vi "ZK HAL.vi"(11 "Interface":T1={"SYSTEM Interface"={"运行模式"=enum."维护模式", "站点类型"=enum."一体站", "CODMn类型"=enum."PLC版", "总磷总氮类型"=enum."单模块", "CODcr模块版本"=enum."斯坦道V3", "性能测试模式"=FALSE}, "Pump Interface"={"Pump MB session in"=refnum}, "NH3N Interface"={"NH3N session in"=refnum, "氨氮自动测试量程配置"={"水样测试量程模式"=enum."AUTO", "空白核查量程模式"=enum."AUTO", "跨度核查量程模式"=enum."AUTO", "加标回收量程模式"=enum."AUTO"}, "命令格式"=0}, "TP Interface"={"TP MB session in"=refnum, "总磷自动测试量程配置"={"水样测试量程模式"=enum."AUTO", "空白核查量程模式"=enum."AUTO", "跨度核查量程模式"=enum."AUTO", "加标回收量程模式"=enum."AUTO"}, "命令格式"=0}, "TN Interface"={"TN MB session in"=refnum, "总氮自动测试量程配置"={"水样测试量程模式"=enum."AUTO", "空白核查量程模式"=enum."AUTO", "跨度核查量程模式"=enum."AUTO", "加标回收量程模式"=enum."AUTO"}, "命令格式"=0}, "CODMn Interface"={"CODMn MB session in"=refnum, "CODMn自动测试量程配置"={"水样测试量程模式"=enum."AUTO", "空白核查量程模式"=enum."AUTO", "跨度核查量程模式"=enum."AUTO", "加标回收量程模式"=enum."AUTO"}, "命令格式"=0}, "CODCr Interface"={"CODCr MB session in"=refnum, "CODCr自动测试量程配置"={"水样测试量程模式"=enum."AUTO", "空白核查量程模式"=enum."AUTO", "跨度核查量程模式"=enum."AUTO", "加标回收量程模式"=enum."AUTO"}, "命令格式"=0}, "PLC_CODMn Interface"={"PLC版_CODMn状态"=0, "PLC版_CODMn测量数据区"={"因子编码"=0, "单位"=0, "标样参考值"=0.0, "水样数据时间"=timestamp(0 s since 1904-01-01), "水样实测值"=0.0, "水样数据标识"="", "标样数据时间"=timestamp(0 s since 1904-01-01), "标样实测值"=0.0, "标样数据标识"="", "空白数据时间"=timestamp(0 s since 1904-01-01), "空白实测值"=0.0, "空白数据标识"="", "零点核查数据时间"=timestamp(0 s since 1904-01-01), "零点核查实测值"=0.0, "零点核查数据标识"="", "跨度核查数据时间"=timestamp(0 s since 1904-01-01), "跨度核查实测值"=0.0, "跨度核查数据标识"="", "加标回收数据时间"=timestamp(0 s since 1904-01-01), "加标回收实测值"=0.0, "加标回收数据标识"="", "平行样数据时间"=timestamp(0 s since 1904-01-01), "平行样实测值"=0.0, "平行样数据标识"=""}}, "氟化物 Interface"={"MB session in"=refnum, "自动测试量程配置"={"水样测试量程模式"=enum."AUTO", "空白核查量程模式"=enum."AUTO", "跨度核查量程模式"=enum."AUTO", "加标回收量程模式"=enum."AUTO"}}, "挥发酚 Interface"={"挥发酚工作状态"=0, "挥发酚 MB session in"=refnum, "挥发酚_测量数据区"={"因子编码"=0, "单位"=0, "标样2参考值"=0.0, "水样数据时间"=timestamp(0 s since 1904-01-01), "水样实测值"=0.0, "水样数据标识"="", "标样2数据时间"=timestamp(0 s since 1904-01-01), "标样2实测值"=0.0, "标样2数据标识"="", "空白数据时间"=timestamp(0 s since 1904-01-01), "空白实测值"=0.0, "空白数据标识"="", "零点核查数据时间"=timestamp(0 s since 1904-01-01), "零点核查实测值"=0.0, "零点核查数据标识"="", "跨度核查数据时间"=timestamp(0 s since 1904-01-01), "跨度核查实测值"=0.0, "跨度核查数据标识"="", "加标回收数据时间"=timestamp(0 s since 1904-01-01), "加标回收实测值"=0.0, "加标回收数据标识"="", "平行样数据时间"=timestamp(0 s since 1904-01-01), "平行样实测值"=0.0, "平行样数据标识"="", "标样1参考值"=0.0, "标样1数据时间"=timestamp(0 s since 1904-01-01), "标样1实测值"=0.0, "标样1数据标识"="", "标样核查数据时间"=timestamp(0 s since 1904-01-01), "标样核查实测值"=0.0, "标样核查数据标识"=""}}} {"挥发酚 Interface"."挥发酚_测量数据区"."单位" items=["ug/L", "mg/L", "ppm", "mg/m3", "cm", "ppb", "ug/m3", "%", "nmol/mol", "umol/mol", "MPN/L", "MPN/100ml", "ng/m3", "NTU", "无量纲", "ms/cm", "us/cm", "℃", "mV", "万个/L"]; "挥发酚 Interface"."挥发酚工作状态" items=["空闲"=0, "水样测试"=1, "标样核查"=2, "零点核查"=3, "跨度核查"=4, "空白测试"=5, "平行样测试"=6, "加标回收"=7, "空白校准"=8, "标样校准"=9, "标定"=19, "初始化（清洗）"=10, "标样1测量"=28, "标样2测量"=29, "故障"=30, "异常处理"=31, "初始装液"=32, "其他"=33]; "PLC_CODMn Interface"."PLC版_CODMn状态" items=["待机", "润洗", "进样", "加草酸钠", "反滴定", "排液"]; "PLC_CODMn Interface"."PLC版_CODMn测量数据区"."单位" items=["ug/L", "mg/L", "ppm", "mg/m3", "cm", "ppb", "ug/m3", "%", "nmol/mol", "umol/mol", "MPN/L", "MPN/100ml", "ng/m3", "NTU", "无量纲", "ms/cm", "us/cm", "℃", "mV", "万个/L"]; "CODCr Interface"."命令格式" items=["自动", "低位在前", "低位在后"]; "CODMn Interface"."命令格式" items=["自动", "低位在前", "低位在后"]; "TN Interface"."命令格式" items=["自动", "低位在前", "低位在后"]; "TP Interface"."命令格式" items=["自动", "低位在前", "低位在后"]; "NH3N Interface"."命令格式" items=["自动", "低位在前", "低位在后"]}) -> ()   [LabVIEW 2016]
uses:
  <vilib>/Plasmionique/MB Master/MB_Master/MB_Master.lvclass
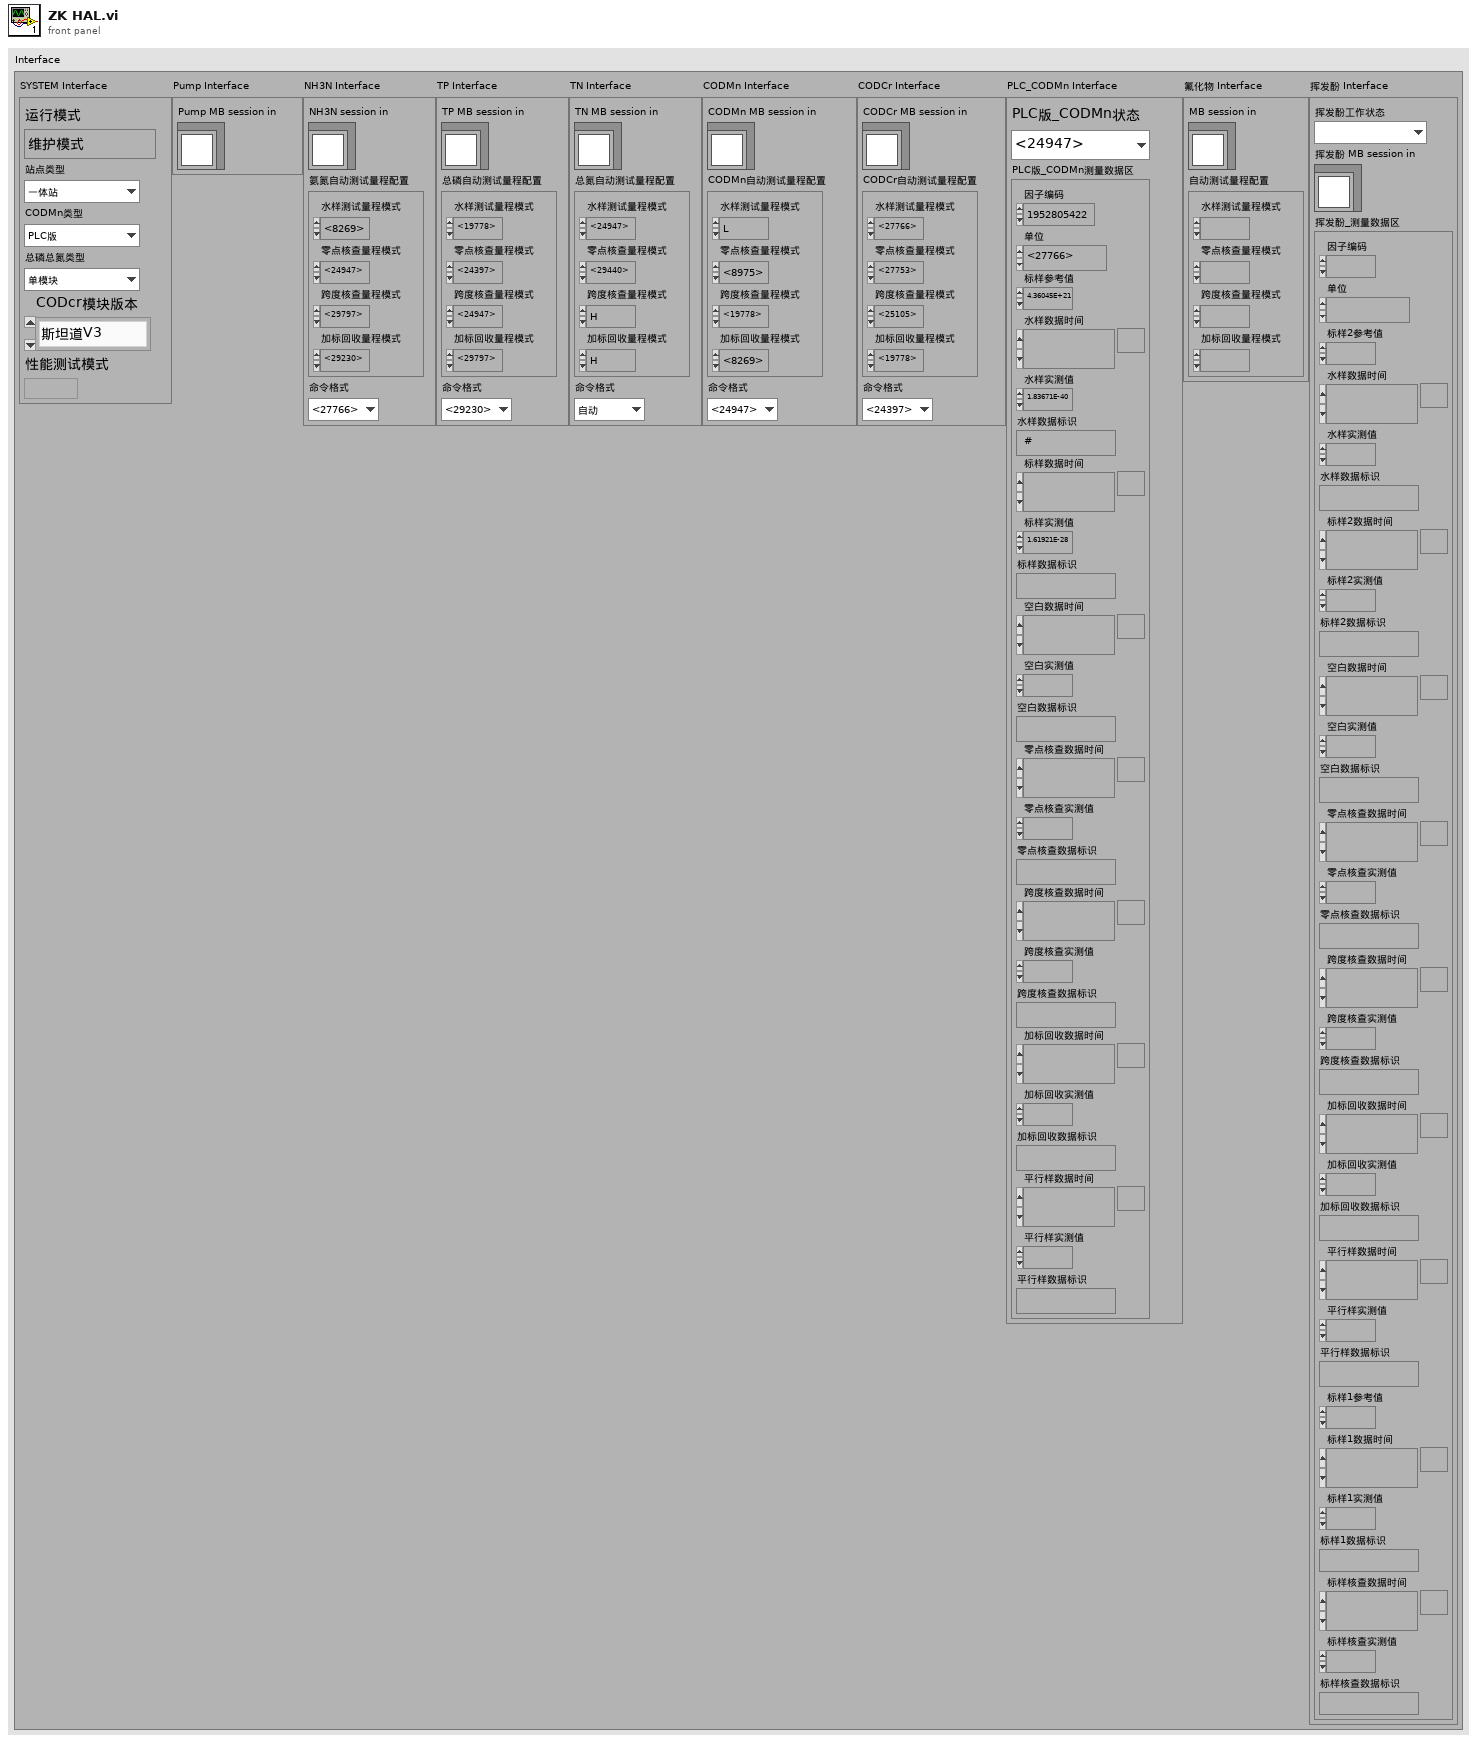
[diagram p1: front panel]
types:
  T1 = cluster{"SYSTEM Interface":cluster{"运行模式":enum16{"维护模式", "常规模式", "应急模式", "质控模式"}, "站点类型":enum16{"一体站", "固定站", "浮船", "一体站V1-V3", "养殖渭水"}, "CODMn类型":enum16{"PLC版", "单片机版"}, "总磷总氮类型":enum16{"单模块", "总磷总氮二合一模块", "氨氮总磷二合一模块"}, "CODcr模块版本":enum16{"斯坦道V3", "点创"}, "性能测试模式":bool}, "Pump Interface":cluster{"Pump MB session in":refnum<class "MB_Master.lvclass">}, "NH3N Interface":cluster{"NH3N session in":refnum<class "MB_Master.lvclass">, "氨氮自动测试量程配置":cluster{"水样测试量程模式":enum16{"H", "L", "AUTO"}, "空白核查量程模式":enum16{"H", "L", "AUTO"}, "跨度核查量程模式":enum16{"H", "L", "AUTO"}, "加标回收量程模式":enum16{"H", "L", "AUTO"}}, "命令格式":u16}, "TP Interface":cluster{"TP MB session in":refnum<class "MB_Master.lvclass">, "总磷自动测试量程配置":cluster{"水样测试量程模式":enum16{"H", "L", "AUTO"}, "空白核查量程模式":enum16{"H", "L", "AUTO"}, "跨度核查量程模式":enum16{"H", "L", "AUTO"}, "加标回收量程模式":enum16{"H", "L", "AUTO"}}, "命令格式":u16}, "TN Interface":cluster{"TN MB session in":refnum<class "MB_Master.lvclass">, "总氮自动测试量程配置":cluster{"水样测试量程模式":enum16{"H", "L", "AUTO"}, "空白核查量程模式":enum16{"H", "L", "AUTO"}, "跨度核查量程模式":enum16{"H", "L", "AUTO"}, "加标回收量程模式":enum16{"H", "L", "AUTO"}}, "命令格式":u16}, "CODMn Interface":cluster{"CODMn MB session in":refnum<class "MB_Master.lvclass">, "CODMn自动测试量程配置":cluster{"水样测试量程模式":enum16{"H", "L", "AUTO"}, "空白核查量程模式":enum16{"H", "L", "AUTO"}, "跨度核查量程模式":enum16{"H", "L", "AUTO"}, "加标回收量程模式":enum16{"H", "L", "AUTO"}}, "命令格式":u16}, "CODCr Interface":cluster{"CODCr MB session in":refnum<class "MB_Master.lvclass">, "CODCr自动测试量程配置":cluster{"水样测试量程模式":enum16{"H", "L", "AUTO"}, "空白核查量程模式":enum16{"H", "L", "AUTO"}, "跨度核查量程模式":enum16{"H", "L", "AUTO"}, "加标回收量程模式":enum16{"H", "L", "AUTO"}}, "命令格式":u16}, "PLC_CODMn Interface":cluster{"PLC版_CODMn状态":u16, "PLC版_CODMn测量数据区":cluster{"因子编码":u32, "单位":u16, "标样参考值":sgl, "水样数据时间":timestamp, "水样实测值":sgl, "水样数据标识":string, "标样数据时间":timestamp, "标样实测值":sgl, "标样数据标识":string, "空白数据时间":timestamp, "空白实测值":sgl, "空白数据标识":string, "零点核查数据时间":timestamp, "零点核查实测值":sgl, "零点核查数据标识":string, "跨度核查数据时间":timestamp, "跨度核查实测值":sgl, "跨度核查数据标识":string, "加标回收数据时间":timestamp, "加标回收实测值":sgl, "加标回收数据标识":string, "平行样数据时间":timestamp, "平行样实测值":sgl, "平行样数据标识":string}}, "氟化物 Interface":cluster{"MB session in":refnum<class "MB_Master.lvclass">, "自动测试量程配置":cluster{"水样测试量程模式":enum16{"H", "L", "AUTO"}, "空白核查量程模式":enum16{"H", "L", "AUTO"}, "跨度核查量程模式":enum16{"H", "L", "AUTO"}, "加标回收量程模式":enum16{"H", "L", "AUTO"}}}, "挥发酚 Interface":cluster{"挥发酚工作状态":u16, "挥发酚 MB session in":refnum<class "MB_Master.lvclass">, "挥发酚_测量数据区":cluster{"因子编码":u32, "单位":u16, "标样2参考值":sgl, "水样数据时间":timestamp, "水样实测值":sgl, "水样数据标识":string, "标样2数据时间":timestamp, "标样2实测值":sgl, "标样2数据标识":string, "空白数据时间":timestamp, "空白实测值":sgl, "空白数据标识":string, "零点核查数据时间":timestamp, "零点核查实测值":sgl, "零点核查数据标识":string, "跨度核查数据时间":timestamp, "跨度核查实测值":sgl, "跨度核查数据标识":string, "加标回收数据时间":timestamp, "加标回收实测值":sgl, "加标回收数据标识":string, "平行样数据时间":timestamp, "平行样实测值":sgl, "平行样数据标识":string, "标样1参考值":sgl, "标样1数据时间":timestamp, "标样1实测值":sgl, "标样1数据标识":string, "标样核查数据时间":timestamp, "标样核查实测值":sgl, "标样核查数据标识":string}}}
  T2 = cluster{"运行模式":enum16{"维护模式", "常规模式", "应急模式", "质控模式"}, "站点类型":enum16{"一体站", "固定站", "浮船", "一体站V1-V3", "养殖渭水"}, "CODMn类型":enum16{"PLC版", "单片机版"}, "总磷总氮类型":enum16{"单模块", "总磷总氮二合一模块", "氨氮总磷二合一模块"}, "CODcr模块版本":enum16{"斯坦道V3", "点创"}, "性能测试模式":bool}
  T3 = cluster{"Pump MB session in":refnum<class "MB_Master.lvclass">}
  T4 = cluster{"NH3N session in":refnum<class "MB_Master.lvclass">, "氨氮自动测试量程配置":cluster{"水样测试量程模式":enum16{"H", "L", "AUTO"}, "空白核查量程模式":enum16{"H", "L", "AUTO"}, "跨度核查量程模式":enum16{"H", "L", "AUTO"}, "加标回收量程模式":enum16{"H", "L", "AUTO"}}, "命令格式":u16}
  T5 = cluster{"TP MB session in":refnum<class "MB_Master.lvclass">, "总磷自动测试量程配置":cluster{"水样测试量程模式":enum16{"H", "L", "AUTO"}, "空白核查量程模式":enum16{"H", "L", "AUTO"}, "跨度核查量程模式":enum16{"H", "L", "AUTO"}, "加标回收量程模式":enum16{"H", "L", "AUTO"}}, "命令格式":u16}
  T6 = cluster{"TN MB session in":refnum<class "MB_Master.lvclass">, "总氮自动测试量程配置":cluster{"水样测试量程模式":enum16{"H", "L", "AUTO"}, "空白核查量程模式":enum16{"H", "L", "AUTO"}, "跨度核查量程模式":enum16{"H", "L", "AUTO"}, "加标回收量程模式":enum16{"H", "L", "AUTO"}}, "命令格式":u16}
  T7 = cluster{"CODMn MB session in":refnum<class "MB_Master.lvclass">, "CODMn自动测试量程配置":cluster{"水样测试量程模式":enum16{"H", "L", "AUTO"}, "空白核查量程模式":enum16{"H", "L", "AUTO"}, "跨度核查量程模式":enum16{"H", "L", "AUTO"}, "加标回收量程模式":enum16{"H", "L", "AUTO"}}, "命令格式":u16}
  T8 = cluster{"CODCr MB session in":refnum<class "MB_Master.lvclass">, "CODCr自动测试量程配置":cluster{"水样测试量程模式":enum16{"H", "L", "AUTO"}, "空白核查量程模式":enum16{"H", "L", "AUTO"}, "跨度核查量程模式":enum16{"H", "L", "AUTO"}, "加标回收量程模式":enum16{"H", "L", "AUTO"}}, "命令格式":u16}
  T9 = cluster{"PLC版_CODMn状态":u16, "PLC版_CODMn测量数据区":cluster{"因子编码":u32, "单位":u16, "标样参考值":sgl, "水样数据时间":timestamp, "水样实测值":sgl, "水样数据标识":string, "标样数据时间":timestamp, "标样实测值":sgl, "标样数据标识":string, "空白数据时间":timestamp, "空白实测值":sgl, "空白数据标识":string, "零点核查数据时间":timestamp, "零点核查实测值":sgl, "零点核查数据标识":string, "跨度核查数据时间":timestamp, "跨度核查实测值":sgl, "跨度核查数据标识":string, "加标回收数据时间":timestamp, "加标回收实测值":sgl, "加标回收数据标识":string, "平行样数据时间":timestamp, "平行样实测值":sgl, "平行样数据标识":string}}
  T10 = cluster{"MB session in":refnum<class "MB_Master.lvclass">, "自动测试量程配置":cluster{"水样测试量程模式":enum16{"H", "L", "AUTO"}, "空白核查量程模式":enum16{"H", "L", "AUTO"}, "跨度核查量程模式":enum16{"H", "L", "AUTO"}, "加标回收量程模式":enum16{"H", "L", "AUTO"}}}
  T11 = cluster{"挥发酚工作状态":u16, "挥发酚 MB session in":refnum<class "MB_Master.lvclass">, "挥发酚_测量数据区":cluster{"因子编码":u32, "单位":u16, "标样2参考值":sgl, "水样数据时间":timestamp, "水样实测值":sgl, "水样数据标识":string, "标样2数据时间":timestamp, "标样2实测值":sgl, "标样2数据标识":string, "空白数据时间":timestamp, "空白实测值":sgl, "空白数据标识":string, "零点核查数据时间":timestamp, "零点核查实测值":sgl, "零点核查数据标识":string, "跨度核查数据时间":timestamp, "跨度核查实测值":sgl, "跨度核查数据标识":string, "加标回收数据时间":timestamp, "加标回收实测值":sgl, "加标回收数据标识":string, "平行样数据时间":timestamp, "平行样实测值":sgl, "平行样数据标识":string, "标样1参考值":sgl, "标样1数据时间":timestamp, "标样1实测值":sgl, "标样1数据标识":string, "标样核查数据时间":timestamp, "标样核查实测值":sgl, "标样核查数据标识":string}}
  T12 = cluster{"因子编码":u32, "单位":u16, "标样参考值":sgl, "水样数据时间":timestamp, "水样实测值":sgl, "水样数据标识":string, "标样数据时间":timestamp, "标样实测值":sgl, "标样数据标识":string, "空白数据时间":timestamp, "空白实测值":sgl, "空白数据标识":string, "零点核查数据时间":timestamp, "零点核查实测值":sgl, "零点核查数据标识":string, "跨度核查数据时间":timestamp, "跨度核查实测值":sgl, "跨度核查数据标识":string, "加标回收数据时间":timestamp, "加标回收实测值":sgl, "加标回收数据标识":string, "平行样数据时间":timestamp, "平行样实测值":sgl, "平行样数据标识":string}
  T13 = cluster{"水样测试量程模式":enum16{"H", "L", "AUTO"}, "空白核查量程模式":enum16{"H", "L", "AUTO"}, "跨度核查量程模式":enum16{"H", "L", "AUTO"}, "加标回收量程模式":enum16{"H", "L", "AUTO"}}
  T14 = cluster{"因子编码":u32, "单位":u16, "标样2参考值":sgl, "水样数据时间":timestamp, "水样实测值":sgl, "水样数据标识":string, "标样2数据时间":timestamp, "标样2实测值":sgl, "标样2数据标识":string, "空白数据时间":timestamp, "空白实测值":sgl, "空白数据标识":string, "零点核查数据时间":timestamp, "零点核查实测值":sgl, "零点核查数据标识":string, "跨度核查数据时间":timestamp, "跨度核查实测值":sgl, "跨度核查数据标识":string, "加标回收数据时间":timestamp, "加标回收实测值":sgl, "加标回收数据标识":string, "平行样数据时间":timestamp, "平行样实测值":sgl, "平行样数据标识":string, "标样1参考值":sgl, "标样1数据时间":timestamp, "标样1实测值":sgl, "标样1数据标识":string, "标样核查数据时间":timestamp, "标样核查实测值":sgl, "标样核查数据标识":string}
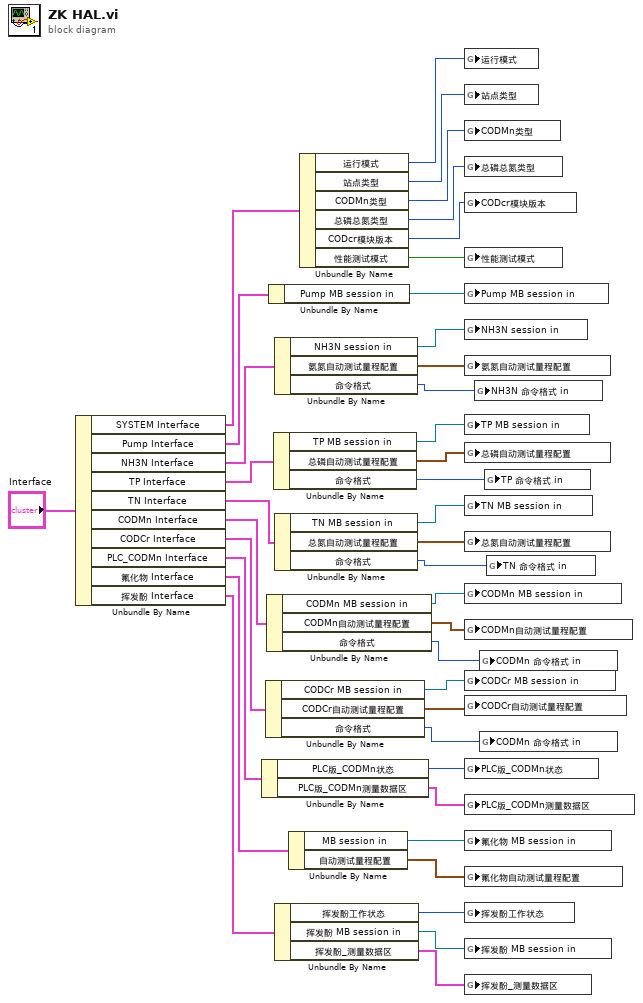
[diagram p0: block diagram]
diagram:
  n1 = Unbundle By Name("Interface") -> ("SYSTEM Interface"=w39:T2, "Pump Interface"=w37:T3, "NH3N Interface"=w35:T4, "TP Interface"=w32:T5, "TN Interface"=w29:T6, "CODMn Interface"=w26:T7, "CODCr Interface"=w23:T8, "PLC_CODMn Interface"=w20:T9, "氟化物 Interface"=w14:T10, "挥发酚 Interface"=w10:T11)
  n2 = Unbundle By Name(w20) -> ("PLC版_CODMn状态"=w19:u16, "PLC版_CODMn测量数据区"=w18:T12)
  n3 = Unbundle By Name(w23) -> ("CODCr MB session in"=w22:refnum<class "MB_Master.lvclass">, "CODCr自动测试量程配置"=w21:T13, "命令格式"=w5:u16)
  n4 = Unbundle By Name(w26) -> ("CODMn MB session in"=w25:refnum<class "MB_Master.lvclass">, "CODMn自动测试量程配置"=w24:T13, "命令格式"=w4:u16)
  n5 = Unbundle By Name(w37) -> ("Pump MB session in"=w36:refnum<class "MB_Master.lvclass">)
  n6 = Unbundle By Name(w32) -> ("TP MB session in"=w31:refnum<class "MB_Master.lvclass">, "总磷自动测试量程配置"=w30:T13, "命令格式"=w2:u16)
  n7 = Unbundle By Name(w35) -> ("NH3N session in"=w33:refnum<class "MB_Master.lvclass">, "氨氮自动测试量程配置"=w34:T13, "命令格式"=w1:u16)
  n8 = Unbundle By Name(w29) -> ("TN MB session in"=w28:refnum<class "MB_Master.lvclass">, "总氮自动测试量程配置"=w27:T13, "命令格式"=w3:u16)
  n9 = Unbundle By Name(w10) -> ("挥发酚工作状态"=w9:u16, "挥发酚 MB session in"=w8:refnum<class "MB_Master.lvclass">, "挥发酚_测量数据区"=w7:T14)
  n10 = Unbundle By Name(w14) -> ("MB session in"=w13:refnum<class "MB_Master.lvclass">, "自动测试量程配置"=w12:T13)
  n11 = Unbundle By Name(w39) -> ("运行模式"=w38:enum16{"维护模式", "常规模式", "应急模式", "质控模式"}, "站点类型"=w16:enum16{"一体站", "固定站", "浮船", "一体站V1-V3", "养殖渭水"}, "CODMn类型"=w17:enum16{"PLC版", "单片机版"}, "总磷总氮类型"=w15:enum16{"单模块", "总磷总氮二合一模块", "氨氮总磷二合一模块"}, "CODcr模块版本"=w11:enum16{"斯坦道V3", "点创"}, "性能测试模式"=w6:bool)
  n12 = global write "系统交互.vi" "运行模式"(w38) -> ()
  n13 = global write "系统交互.vi" "站点类型"(w16) -> ()
  n14 = global write "系统交互.vi" "CODMn类型"(w17) -> ()
  n15 = global write "系统交互.vi" "总磷总氮类型"(w15) -> ()
  n16 = global write "系统交互.vi" "CODcr模块版本"(w11) -> ()
  n17 = global write "系统交互.vi" "性能测试模式"(w6) -> ()
  n18 = global write "系统交互.vi" "Pump MB session in"(w36) -> ()
  n19 = global write "系统交互.vi" "NH3N session in"(w33) -> ()
  n20 = global write "系统交互.vi" "氨氮自动测试量程配置"(w34) -> ()
  n21 = global write "系统交互.vi" "TP MB session in"(w31) -> ()
  n22 = global write "系统交互.vi" "总磷自动测试量程配置"(w30) -> ()
  n23 = global write "系统交互.vi" "TN MB session in"(w28) -> ()
  n24 = global write "系统交互.vi" "总氮自动测试量程配置"(w27) -> ()
  n25 = global write "系统交互.vi" "CODMn MB session in"(w25) -> ()
  n26 = global write "系统交互.vi" "CODMn自动测试量程配置"(w24) -> ()
  n27 = global write "系统交互.vi" "CODCr MB session in"(w22) -> ()
  n28 = global write "系统交互.vi" "CODCr自动测试量程配置"(w21) -> ()
  n29 = global write "系统交互.vi" "PLC版_CODMn状态"(w19) -> ()
  n30 = global write "系统交互.vi" "PLC版_CODMn测量数据区"(w18) -> ()
  n31 = global write "系统交互.vi" "氟化物 MB session in"(w13) -> ()
  n32 = global write "系统交互.vi" "氟化物自动测试量程配置"(w12) -> ()
  n33 = global write "系统交互.vi" "挥发酚工作状态"(w9) -> ()
  n34 = global write "系统交互.vi" "挥发酚 MB session in"(w8) -> ()
  n35 = global write "系统交互.vi" "挥发酚_测量数据区"(w7) -> ()
  n36 = global write "系统交互.vi" "NH3N 命令格式 in"(w1) -> ()
  n37 = global write "系统交互.vi" "CODMn 命令格式 in"(w4) -> ()
  n38 = global write "系统交互.vi" "CODMn 命令格式 in"(w5) -> ()
  n39 = global write "系统交互.vi" "TP 命令格式 in"(w2) -> ()
  n40 = global write "系统交互.vi" "TN 命令格式 in"(w3) -> ()
